vi "Theta 2.vi"(8 "XYZ_60":dbl[](array[numeric])=[0.0, 0.0, 0.0], 9 "XYZ_0":dbl[](array[numeric])=[0.0, 0.0, 0.0], 10 "theta_0":dbl, 11 "6R Type 1 Serial Arm Class in":refnum<class "NI_Robotics_6R Type 1 Serial Arm Class.lvclass">) -> (1 "Valid":bool, 2 "theta_2 array":dbl[](array[numeric]), 3 "6R Type 1 Serial Arm Class out":refnum<class "NI_Robotics_6R Type 1 Serial Arm Class.lvclass">)   [LabVIEW 2017, in "NI_Robotics_6R Type 1 Serial Arm Class.lvclass"]
uses:
  <vilib>/robotics/Kinematics/Analytical/6R/Type 1/NI_Robotics_6R Type 1 Serial Arm Class.lvclass
  c:/Program Files (x86)/National Instruments/LabVIEW 2017/vi.lib/robotics/Kinematics/Analytical/Generic/NI_Robotics_Analytical Serial Arm Class.lvclass
  <vilib>/robotics/Kinematics/Analytical/NI_Robotics_AnalyticKinematics.lvlib
  <vilib>/robotics/Kinematics/Analytical/Generic/NI_Robotics_Analytical Serial Arm Class.lvclass
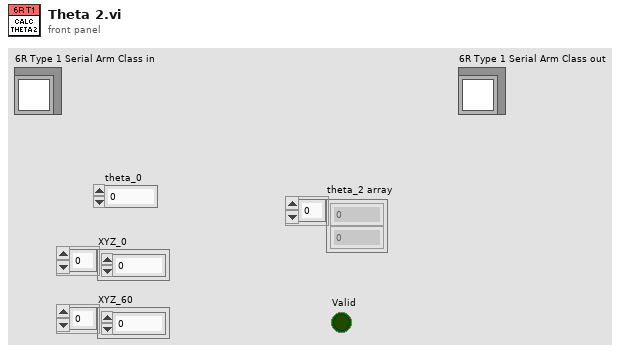
[diagram p1: front panel]
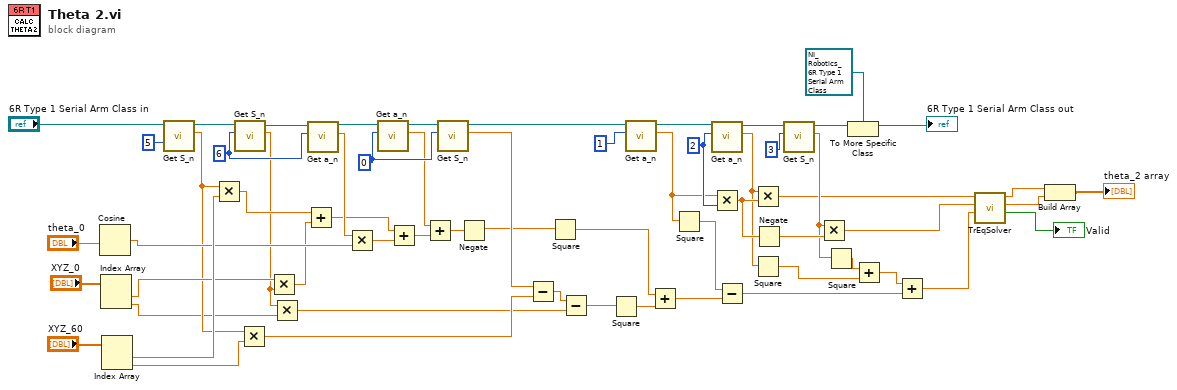
[diagram p0: block diagram]
diagram:
  w26 = 2 ("n")
  w54 = 0 ("n")
  w57 = 6 ("n")
  n1 = Cosine(x="theta_0") -> (cos(x)=w44:dbl)
  n2 = Index Array(array="XYZ_0") -> (element #1=w49:dbl, element #2=w34:dbl)  [unwired: 2 in]
  n3 = Index Array(array="XYZ_60") -> (element #1=w51:dbl, element #2=w37:dbl)  [unwired: 2 in]
  n4 = call <vilib>:"Get S_n.vi"("n"=5, "Analytical Serial Arm Class in"="6R Type 1 Serial Arm Class in") -> ("S_n"=w38:dbl, "Analytical Serial Arm Class out"=w60:refnum<class "NI_Robotics_6R Type 1 Serial Arm Class.lvclass">)  [unwired: 8 in]
  n5 = Multiply(x=w38, y=w51) -> (x*y=w50:dbl)
  n6 = call <vilib>:"Get S_n.vi"("n"=w57, "Analytical Serial Arm Class in"=w60) -> ("S_n"=w35:dbl, "Analytical Serial Arm Class out"=w58:refnum<class "NI_Robotics_6R Type 1 Serial Arm Class.lvclass">)  [unwired: 8 in]
  n7 = Multiply(x=w38, y=w37) -> (x*y=w36:dbl)
  n8 = Multiply(x=w49, y=w35) -> (x*y=w43:dbl)
  n9 = Multiply(x=w35, y=w34) -> (x*y=w32:dbl)
  n10 = Add(x=w50, y=w43) -> (x+y=w45:dbl)
  n11 = call <vilib>:"Get a_n.vi"("n"=w57, "Analytical Serial Arm Class in"=w58) -> ("a_n"=w47:dbl, "Analytical Serial Arm Class out"=w56:refnum<class "NI_Robotics_6R Type 1 Serial Arm Class.lvclass">)  [unwired: 8 in]
  n12 = Multiply(x=w47, y=w44) -> (x*y=w46:dbl)
  n13 = call <vilib>:"Get a_n.vi"("n"=w54, "Analytical Serial Arm Class in"=w56) -> ("a_n"=w41:dbl, "Analytical Serial Arm Class out"=w55:refnum<class "NI_Robotics_6R Type 1 Serial Arm Class.lvclass">)  [unwired: 8 in]
  n14 = Add(x=w45, y=w46) -> (x+y=w42:dbl)
  n15 = Add(x=w41, y=w42) -> (x+y=w40:dbl)
  n16 = call <vilib>:"Get S_n.vi"("n"=w54, "Analytical Serial Arm Class in"=w55) -> ("S_n"=w39:dbl, "Analytical Serial Arm Class out"=w30:refnum<class "NI_Robotics_6R Type 1 Serial Arm Class.lvclass">)  [unwired: 8 in]
  n17 = Negate(x=w40) -> (-x=w23:dbl)
  n18 = Subtract(x=w39, y=w36) -> (x-y=w33:dbl)
  n19 = Square(x=w23) -> (x^2=w20:dbl)
  n20 = Subtract(x=w33, y=w32) -> (x-y=w22:dbl)
  n21 = Square(x=w22) -> (x^2=w21:dbl)
  n22 = call <vilib>:"Get a_n.vi"("n"=1, "Analytical Serial Arm Class in"=w30) -> ("a_n"=w19:dbl, "Analytical Serial Arm Class out"=w31:refnum<class "NI_Robotics_6R Type 1 Serial Arm Class.lvclass">)  [unwired: 8 in]
  n23 = Add(x=w20, y=w21) -> (x+y=w15:dbl)
  n24 = Square(x=w19) -> (x^2=w16:dbl)
  n25 = call <vilib>:"Get a_n.vi"("n"=w26, "Analytical Serial Arm Class in"=w31) -> ("a_n"=w18:dbl, "Analytical Serial Arm Class out"=w28:refnum<class "NI_Robotics_6R Type 1 Serial Arm Class.lvclass">)  [unwired: 8 in]
  n26 = Multiply(x=w19, y=w26) -> (x*y=w25:dbl)
  n27 = Subtract(x=w16, y=w15) -> (x-y=w11:dbl)
  n28 = Multiply(x=w18, y=w25) -> (x*y=w10:dbl)
  n29 = Square(x=w18) -> (x^2=w17:dbl)
  n30 = Negate(x=w25) -> (-x=w24:dbl)
  n31 = call <vilib>:"Get S_n.vi"("n"=3, "Analytical Serial Arm Class in"=w28) -> ("S_n"=w13:dbl, "Analytical Serial Arm Class out"=w3:refnum<class "NI_Robotics_6R Type 1 Serial Arm Class.lvclass">)  [unwired: 8 in]
  n32 = Multiply(x=w13, y=w24) -> (x*y=w9:dbl)
  n33 = Square(x=w13) -> (x^2=w14:dbl)
  n34 = To More Specific Class(target class=refnum<class "NI_Robotics_6R Type 1 Serial Arm Class.lvclass"> refnum ("6R Type 1 Serial Arm Class in"), reference=w3) -> (specific class reference=→"6R Type 1 Serial Arm Class out":refnum<class "NI_Robotics_6R Type 1 Serial Arm Class.lvclass">)  [unwired: 1 in, 1 out]
  n35 = Add(x=w14, y=w17) -> (x+y=w12:dbl)
  n36 = Add(x=w12, y=w11) -> (x+y=w8:dbl)
  n37 = call <vilib>:"TrEqSolver.vi"("D"=w8, "B"=w9, "A"=w10) -> ("Solution Exists"=→"Valid":bool, "angle 2"=w6:dbl, "angle 1"=w5:dbl)  [unwired: 6 in]
  n38 = Build Array(w5, w6) -> (→"theta_2 array":dbl[])
